vi "set_position_cursor.vi"(8 "error in (no error)":errorcluster, 9 "raw channel index":i32, 11 "DisplayDL090216 in":refnum<class "DisplayDL090216.lvclass">) -> (0 "error out":errorcluster, 3 "DisplayDL090216 out":refnum<class "DisplayDL090216.lvclass">)   [LabVIEW 2010, in "DisplayDL090216.lvclass"]
uses:
  DisplayDL090216.lvclass
  DisplayDL090216.lvclass/DisplayDL090216.ctl
  common/classes/ColorOverlay/ColorOverlay/ColorOverlay.lvclass
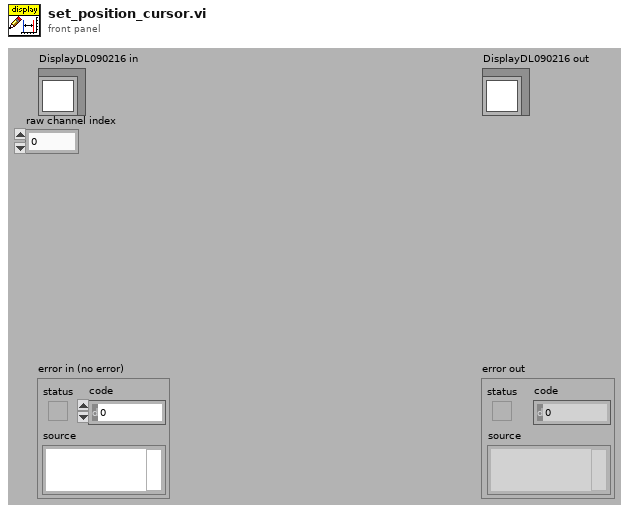
[diagram p1: front panel]
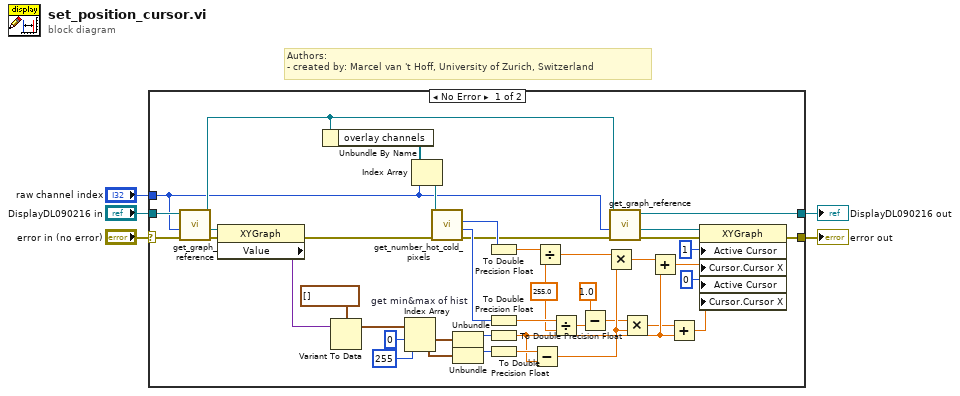
[diagram p0: block diagram]
diagram:
  # "Authors: \n- created by: Marcel van 't Hoff, University of Zurich, Switzerland"
  n1 = case shown="No Error" "error in (no error)" {
    selector: "error in (no error)" -> [w26 w48]
    tunnel: [w19 w48] -> w4
    tunnel: [w23 w47] -> w2
    tunnel: "DisplayDL090216 in" -> [w27 w47]
    tunnel: "raw channel index" -> [w18 _]
    frame No Error {
      w17 = 255.0
      n2 = call-dynamic "get_graph_reference.vi"("error in (no error)"=w26, "raw channel index"=w18, "DisplayDL090216 in"=w27) -> ("error out"=w43:errorcluster, "histogram reference out"=w44:refnum<vi>, "DisplayDL090216 out"=w24:refnum<class "DisplayDL090216.lvclass">)  [unwired: 6 in]
      n3 = property class="XYGraph"(reference=w44, error in=w43) -> (error out=w25:errorcluster, "Value"=w34:variant)  [unwired: 1 out]
      n4 = Unbundle By Name(w24) -> ("overlay channels"=w46:refnum<class "ColorOverlay.lvclass">[])
      n5 = Variant To Data(Variant=w34, type=cluster{i32, u32}[] [] ("histogram out")) -> (data=w35:cluster{i32, u32}[])  [unwired: 1 in, 1 out]
      n6 = Index Array "get min&max of hist"(array=w35, index #1=0 ("index"), index #2=255 ("index")) -> (element #1=w36:cluster{i32, u32}, element #2=w37:cluster{i32, u32})
      n7 = Index Array(array=w46, index=w18) -> (element=w45:refnum<class "ColorOverlay.lvclass">)
      n8 = call-dynamic "get_number_hot_cold_pixels.vi"("error in (no error)"=w25, "ColorOverlay in"=w45) -> ("error out"=w22:errorcluster, "# hot pixels"=w29:i32, "# cold pixels"=w33:i32)  [unwired: 6 in, 1 out]
      n9 = Unbundle(w36) -> (w40:i32)  [unwired: 1 out]
      n10 = Unbundle(w37) -> (w41:i32)  [unwired: 1 out]
      n11 = To Double Precision Float(number=w33) -> (double precision float=w32:dbl)
      n12 = To Double Precision Float(number=w29) -> (double precision float=w28:dbl)
      n13 = To Double Precision Float(number=w40) -> (double precision float=w10:dbl)
      n14 = To Double Precision Float(number=w41) -> (double precision float=w31:dbl)
      n15 = Subtract(x=w31, y=w10) -> (x-y=w16:dbl)
      n16 = Divide(x=w32, y=w17) -> (x/y=w30:dbl)
      n17 = Divide(x=w28, y=w17) -> (x/y=w12:dbl)
      n18 = Subtract(x=1.0, y=w12) -> (x-y=w11:dbl)
      n19 = Multiply(x=w30, y=w16) -> (x*y=w15:dbl)
      n20 = call-dynamic "get_graph_reference.vi"("error in (no error)"=w22, "raw channel index"=w18, "DisplayDL090216 in"=w24) -> ("error out"=w20:errorcluster, "histogram reference out"=w21:refnum<vi>, "DisplayDL090216 out"=w23:refnum<class "DisplayDL090216.lvclass">)  [unwired: 6 in]
      n21 = Multiply(x=w11, y=w16) -> (x*y=w9:dbl)
      n22 = Add(x=w15, y=w10) -> (x+y=w14:dbl)
      n23 = Add(x=w9, y=w10) -> (x+y=w8:dbl)
      n24 = property class="XYGraph"(reference=w21, error in=w20, "Active Cursor"=u32 1, "Cursor.Cursor X"=w14, "Active Cursor"=u32 0, "Cursor.Cursor X"=w8) -> (error out=w19:errorcluster)  [unwired: 1 out]
    }
    frame Error {
    }
  }
  "error out" <- w4
  "DisplayDL090216 out" <- w2
